vi "coal workers safety.vi"() -> ()   [LabVIEW 2022 SP3]
uses:
  <vilib>/MakerHub/LINX/LMH-LINX.lvlib
  <vilib>/MakerHub/LINX/Public/Peripherals/Analog/Analog Read 1 Chan.vi
  <vilib>/MakerHub/LINX/Public/Utilities/Open Serial.vi
  <vilib>/MakerHub/LINX/Public/Peripherals/Digital/Digital Write 1 Chan.vi
panel:
  out "temp":dbl
  out "Gauge":dbl(knob) scale=0.0..100.0
  in  "stop":bool
  in  "ppm":u8
  out "ppm":bool
  in  "humidity":u8
  out "humidity":bool
  in  "temp":u8
  out "temp":bool
  in  "MQ-9":u8
  in  "DHT-22":u8
  in  "Serial Port":refnum<visa-resource-name>="N/A"
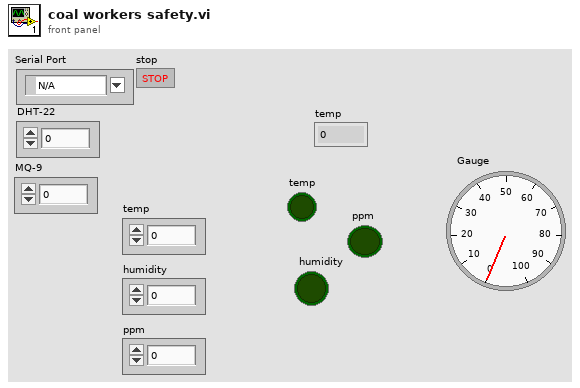
[diagram p1: front panel]
types:
  T1 = typedef "LMH-LINX.lvlib/LINX Ref.ctl" = cluster{"IO":T2, "Interface":T3, "LINX Device Config":T4}
  T2 = typedef "LMH-LINX.lvlib/Platform.ctl" = enum16{"Remote", "Local"}
  T3 = typedef "LMH-LINX.lvlib/Interface.ctl" = enum16{"Serial", "TCP"}
  T4 = typedef "LMH-LINX.lvlib/Device.lvlib/LINX Device Config.ctl" = cluster{"Interface":T3, "COM Port":refnum<visa-resource-name>, "TCP Configuration":T5, "Device Family":u8, "Device ID":u8, "Device Name":string, "TCP Ref":refnum<k5>, "Channels":T6}
  T5 = typedef "LMH-LINX.lvlib/Device.lvlib/TCP Config.ctl" = cluster{"IP Address":string, "Port":u16}
  T6 = typedef "LMH-LINX.lvlib/Channels.ctl" = cluster{"DI":u8[], "DO":u8[], "AI":u8[], "AO":u8[], "PWM":u8[], "QE":u8[], "UART":u8[], "I2C 2":u8[], "SPI":u8[], "CAN":u8[], "Servo":u8[], "AI Ref (V)":dbl, "AI Resolution (Bits)":u8, "AO Ref (V)":dbl, "AO Resolution (Bits)":u8}
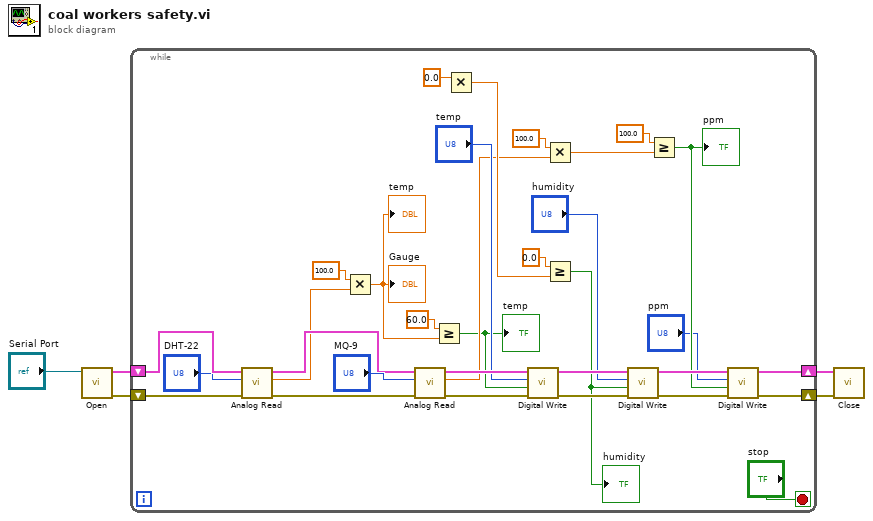
[diagram p0: block diagram]
diagram:
  n1 = call-poly <vilib>:"Open.vi"("Serial Port"="Serial Port") -> ("Error Out"=w2:errorcluster, "LINX Resource"=w4:T1)  [unwired: 8 in, 1 out]
  n2 = while {
    shift-right: [w28] -> w3
    shift-left: w4 -> [w11]
    shift-right: [w27] -> w1
    shift-left: w2 -> [w8]
    stop <- "stop" stop-if-true
    n3 = call-poly <vilib>:"Analog Read.vi"("Error In"=w8, "Analog Channel"="DHT-22", "LINX Resource"=w11) -> ("Error Out"=w9:errorcluster, "Voltage"=w6:dbl, "LINX Resource"=w10:T1)  [unwired: 5 in, 1 out]
    n4 = Multiply(x=100.0, y=w6) -> (x*y=w12:dbl)
    "Gauge" <- w12
    "temp" <- w12
    n5 = call-poly <vilib>:"Analog Read.vi"("Error In"=w9, "Analog Channel"="MQ-9", "LINX Resource"=w10) -> ("Error Out"=w33:errorcluster, "Voltage"=w20:dbl, "LINX Resource"=w34:T1)  [unwired: 5 in, 1 out]
    n6 = Greater Or Equal?(x=60.0, y=w12) -> (x >= y?=w13:bool)
    "temp" <- w13
    n7 = Multiply(x=0.0) -> (x*y=w24:dbl)  [unwired: 1 in]
    n8 = call-poly <vilib>:"Digital Write.vi"("Error In"=w33, "Output Value"=w13, "DO Channel"="temp", "LINX Resource"=w34) -> ("Error Out"=w31:errorcluster, "LINX Resource"=w32:T1)  [unwired: 6 in]
    n9 = Multiply(x=100.0, y=w20) -> (x*y=w18:dbl)
    n10 = Greater Or Equal?(x=0.0, y=w24) -> (x >= y?=w22:bool)
    "humidity" <- w22
    n11 = call-poly <vilib>:"Digital Write.vi"("Error In"=w31, "Output Value"=w22, "DO Channel"="humidity", "LINX Resource"=w32) -> ("Error Out"=w29:errorcluster, "LINX Resource"=w30:T1)  [unwired: 6 in]
    n12 = Greater Or Equal?(x=100.0, y=w18) -> (x >= y?=w16:bool)
    "ppm" <- w16
    n13 = call-poly <vilib>:"Digital Write.vi"("Error In"=w29, "Output Value"=w16, "DO Channel"="ppm", "LINX Resource"=w30) -> ("Error Out"=w27:errorcluster, "LINX Resource"=w28:T1)  [unwired: 6 in]
  }
  n14 = call <vilib>:"Close.vi"("Error In"=w1, "LINX Resource"=w3) -> ()  [unwired: 9 in, 1 out]
